vi "IsUnitTestFrameworkInstalled.vi"(8 "error in (no error)":errorcluster) -> (0 "error out":errorcluster, 2 "IsInstalled":bool)   [LabVIEW 2017, in "UnitTestFrameworkToolkit.lvlib"]
doc: "Returns true if the <B>LabVIEW Unit Test Framework</B> is installed on this machine."
uses:
  <vilib>/nisyscfg/Get Installed Components.vi
  UnitTestFrameworkToolkit.lvlib
  <vilib>/nisyscfg/nisyscfg.lvlib
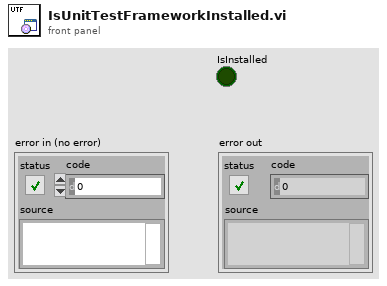
[diagram p1: front panel]
types:
  T1 = typedef "nisyscfg.lvlib/Software 1.2.ctl" = cluster{"title":string, "description":string, "ID":string, "version":string, "component type":T2}
  T2 = typedef "nisyscfg.lvlib/Component Type.ctl" = u32
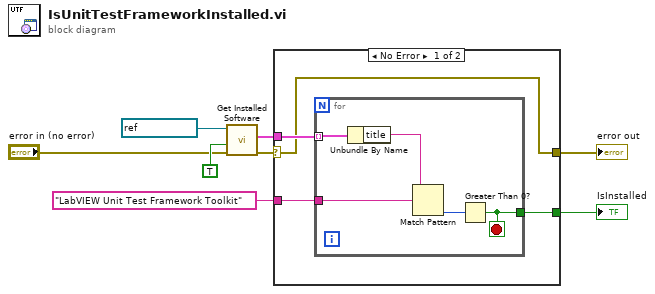
[diagram p0: block diagram]
diagram:
  n1 = call-poly <vilib>:"Get Installed Software.vi"("error in (no error)"="error in (no error)", "Cached (F)"=TRUE, "Session in"=refnum<k21> "localhost") -> ("error out"=w4:errorcluster, "Software Components"=w7:T1[])  [unwired: 6 in, 1 out]
  n2 = case shown="No Error" w4 {
    selector: w4 -> [w9 w18]
    tunnel: w7 -> [w12 _]
    tunnel: "LabVIEW Unit Test Framework Toolkit" ("Component") -> [w11 _]
    tunnel: [w10 _] -> w3
    tunnel: [w9 w18] -> w1
    frame No Error {
      n3 = for {
        tunnel: w12 -> [w17] mode=indexing
        tunnel: w11 -> [w15]
        tunnel: [w13] -> w10
        stop <- w13 stop-if-true
        n4 = Unbundle By Name(w17) -> ("title"=w16:string)
        n5 = Match Pattern(string=w16, regular expression=w15) -> (offset past match=w14:i32)  [unwired: 1 in, 3 out]
        n6 = Greater Than 0?(x=w14) -> (x > 0?=w13:bool)
      }
    }
    frame Error {
    }
  }
  "error out" <- w1
  "IsInstalled" <- w3
